vi "Test - Forward Algorithm.vi"() -> ()   [LabVIEW 2014, in "HMM.lvlib"]
uses:
  HMM.lvlib
panel:
  in  "Scale? (F)":bool
  out "Final Partial Probalility":dbl[][](array[numeric])
  in  "Observed Sequence":i32[](array[numeric])=[0, 2, 3]
  out "Probability":dbl
  in  "HMM Cluster":cluster{"A":dbl[][], "B":dbl[][], "Pi":dbl[]}={"A"=[[0.5, 0.375, 0.125], [0.25, 0.125, 0.625], [0.25, 0.375, 0.375]], "B"=[[0.6, 0.2, 0.15, 0.05], [0.25, 0.25, 0.25, 0.25], [0.05, 0.1, 0.35, 0.5]], "Pi"=[0.63, 0.17, 0.2]}
  # "Expect result: 0.026901"
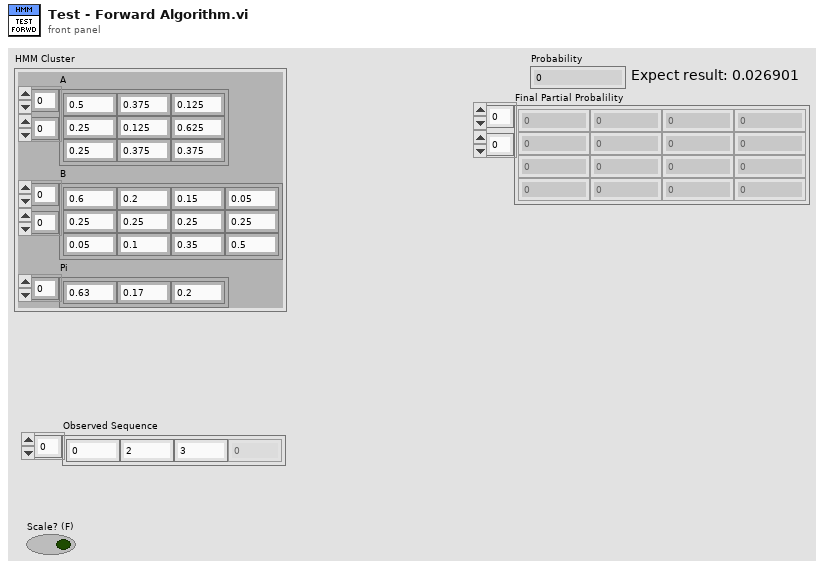
[diagram p1: front panel]
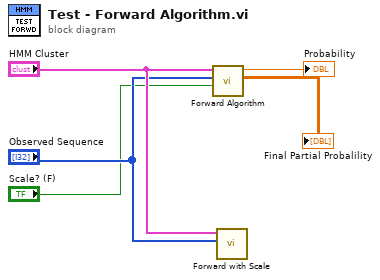
[diagram p0: block diagram]
diagram:
  n1 = call "Forward Algorithm.vi"(9:"Scale? (F)", "O Observed Sequence"="Observed Sequence", "HMM Cluster"="HMM Cluster") -> ("Alpha Partial Probalility"=→"Final Partial Probalility":dbl[][], "Probability"=→"Probability":dbl)  [unwired: 7 in]
  n2 = call "Forward with Scale.vi"("O Observed Sequence"="Observed Sequence", "HMM Cluster"="HMM Cluster") -> ()  [unwired: 7 in, 3 out]
